vi "clearDevice.vi"(8 "error in (no error)":errorcluster, 11 "ElectrometerController in":refnum<class "ElectrometerController.lvclass">) -> (0 "error out":errorcluster, 3 "ElectrometerController out":refnum<class "ElectrometerController.lvclass">)   [LabVIEW 2016, in "ElectrometerController.lvclass"]
uses:
  ElectrometerController.lvclass
  Electrometer/Electrometer.lvclass
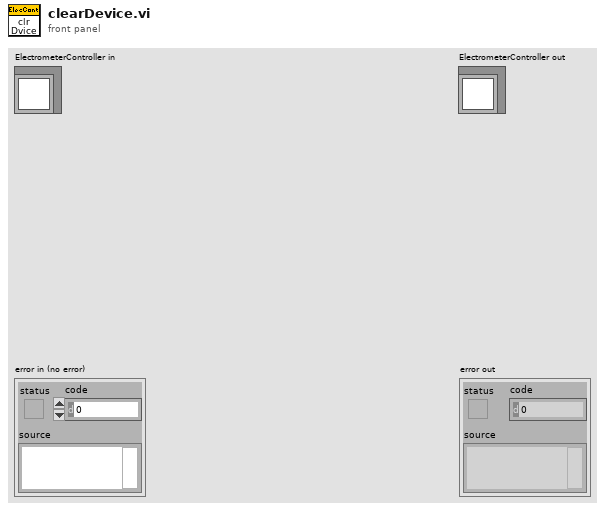
[diagram p1: front panel]
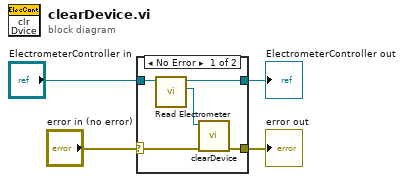
[diagram p0: block diagram]
diagram:
  n1 = case shown="No Error" "error in (no error)" {
    selector: "error in (no error)" -> [w6 w11]
    tunnel: [w5 w11] -> w3
    tunnel: [w8 w10] -> w1
    tunnel: "ElectrometerController in" -> [w9 w10]
    frame No Error {
      n2 = call-dynamic "Read Electrometer.vi"("ElectrometerController in"=w9) -> ("Electrometer.lvclass"=w7:refnum<class "Electrometer.lvclass">, "ElectrometerController out"=w8:refnum<class "ElectrometerController.lvclass">)  [unwired: 8 in, 1 out]
      n3 = call "clearDevice.vi"("error in (no error)"=w6, "Electrometer in"=w7) -> ("error out"=w5:errorcluster)  [unwired: 8 in, 1 out]
    }
    frame Error {
    }
  }
  "error out" <- w3
  "ElectrometerController out" <- w1
